vi "Template.vi"   [LabVIEW 2013]
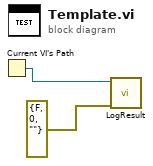
[diagram p0: block diagram]
diagram:
  n1 = Current VI's Path() -> (path=w1:path)
  n2 = call "LogResult.vi"("Test Result"=errorcluster {"status"=FALSE, "code"=0, "source"=""}, "VI Path"=w1) -> ()  [unwired: 10 in]
